vi "Do.vi"(8 "error in (no error)":errorcluster, 10 "Actor in":refnum<class "Actor.lvclass">, 11 "Write and Read VISA Msg":refnum<class "Write and Read VISA Msg.lvclass">) -> (0 "error out":errorcluster, 2 "Actor out":refnum<class "Actor.lvclass">)   [LabVIEW 2020, in "UI ACTOR.lvlib" / "Write and Read VISA Msg.lvclass"]
doc: "This VI delivers the message to the actor by calling the appropriate method(s) on the actor."
uses:
  Write and Read VISA Msg.lvclass
  <vilib>/ActorFramework/Actor/Actor.lvclass
  Write and Read VISA Msg.lvclass/Write and Read VISA Msg.ctl
  UI ACTOR/UI ACTOR.lvclass
  C:/Program Files (x86)/National Instruments/LabVIEW 2020/vi.lib/ActorFramework/Actor/Actor.lvclass
  9ef47adc-f318-494c-9b8b-6df3216d6863.vi
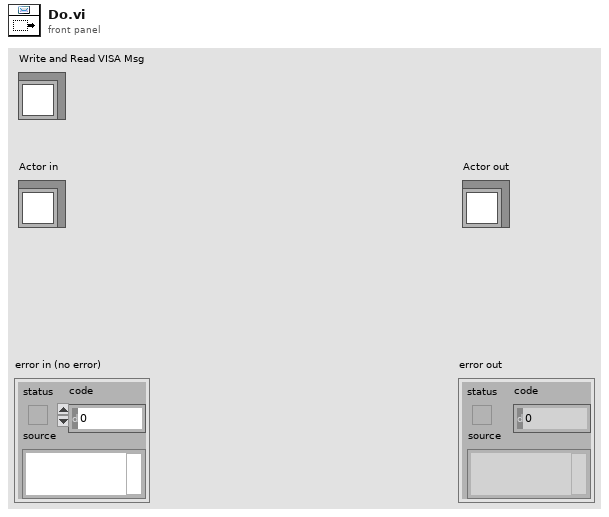
[diagram p1: front panel]
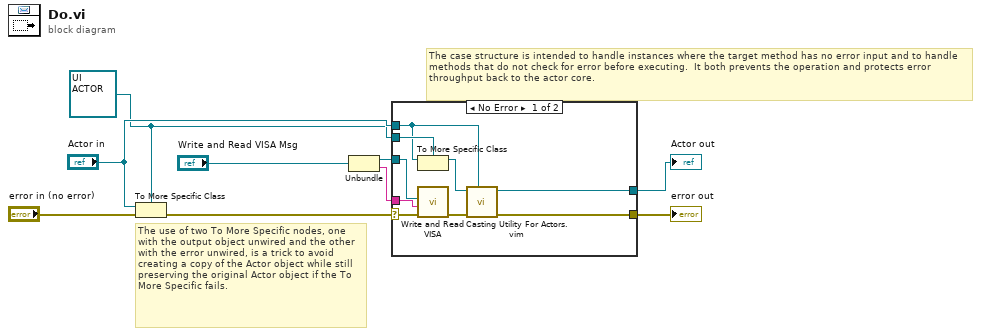
[diagram p0: block diagram]
diagram:
  w3 = refnum<class "UI ACTOR.lvclass"> refnum ("Actor in")
  # "The use of two To More Specific nodes, one with the output object unwired and the other with the error unwired, is a trick to avoid creating a copy of the Actor object while still preserving the original Actor object if the To More Specific fails."
  # "The case structure is intended to handle instances where the target method has no error input and to handle methods that do not check for error before executing.  It both prevents the operation and protects error throughput back to the actor core."
  n1 = To More Specific Class(target class=w3, reference="Actor in", error in="error in (no error)") -> (error out=w7:errorcluster)  [unwired: 1 out]
  n2 = Unbundle("Write and Read VISA Msg") -> (w2:refnum<visa-resource-name>, w1:string)
  n3 = case shown="No Error" w7 {
    selector: w7 -> [w18 w20]
    tunnel: [w13 w20] -> w6
    tunnel: [w14 w19] -> w5
    tunnel: "Actor in" -> [w15 w19]
    tunnel: w3 -> [w16 _]
    tunnel: w2 -> [w11 _]
    tunnel: w1 -> [w10 _]
    frame No Error {
      n4 = To More Specific Class(target class=w16, reference=w15) -> (specific class reference=w17:refnum<class "UI ACTOR.lvclass">)  [unwired: 1 in, 1 out]
      n5 = call "Write and Read VISA.vi"("error in (no error)"=w18, "Command to Send"=w10, "VISA resource name in"=w11) -> ("error out"=w12:errorcluster)  [unwired: 6 in, 2 out]
      n6 = call "Casting Utility For Actors.vim"("type"=w15, "error in (no error)"=w12, "Actor in"=w17) -> ("error out"=w13:errorcluster, "Actor out"=w14:refnum<class "Actor.lvclass">)  [unwired: 7 in]
    }
    frame Error {
      # "If type check fails, pass the original object out again."
    }
  }
  "error out" <- w6
  "Actor out" <- w5
